vi "5302GetOscVoltsVISA.vi"(8 "error in (no error)":errorcluster, 11 "VISA session (for class)":refnum<visa-resource-name>) -> (0 "error out":errorcluster, 1 "data string":string, 2 "Osc Volts":dbl format="%.4f", 3 "VISA session":refnum<visa-resource-name>)   [LabVIEW 2015]
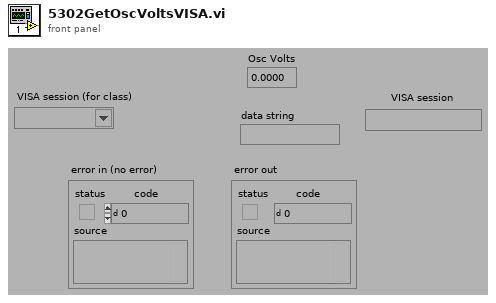
[diagram p1: front panel]
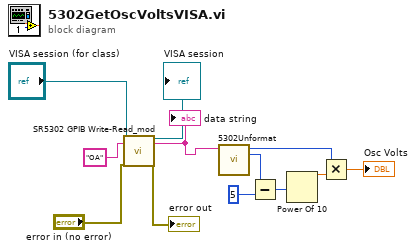
[diagram p0: block diagram]
diagram:
  n1 = call "SR5302 GPIB Write-Read_mod.vi"("VISA session (for class)"="VISA session (for class)", "Write Command String"="OA" ("data string"), "error in (no error)"="error in (no error)") -> ("VISA session"=→"VISA session":refnum<visa-resource-name>, "Response 1"=w1:string, "error out"=→"error out":errorcluster)  [unwired: 5 in, 9 out]
  "data string" <- w1
  n2 = call "5302Unformat.vi"("Data String"=w1) -> ("Numeric 2"=w5:i32, "Numeric 1"=w8:i32)  [unwired: 9 in]
  n3 = Subtract(x=w5, y=5) -> (x-y=w9:i32)
  n4 = Power Of 10(x=w9) -> (10^x=w7:dbl)
  n5 = Multiply(x=w8, y=w7) -> (x*y=→"Osc Volts":dbl)
